vi "Array of params to string.vi"(11 "Array":string[](array[string])) -> (3 "String":string)   [LabVIEW 2019, in "STAV lib.lvlib"]
uses:
  STAV lib.lvlib
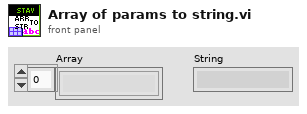
[diagram p1: front panel]
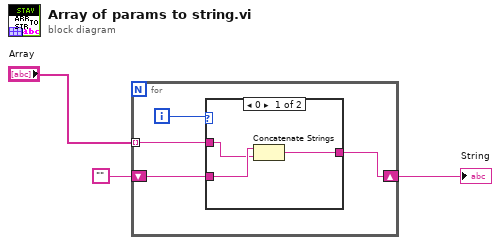
[diagram p0: block diagram]
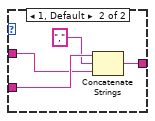
[diagram p2: hidden frame]
diagram:
  n1 = for {
    tunnel: "Array" -> [w6] mode=indexing
    shift-right: [w5] -> w3
    shift-left: "" -> [w7]
    i -> [w4]
    n2 = case shown="0" w4 {
      tunnel: w7 -> [w10 w14]
      tunnel: w6 -> [w9 w13]
      tunnel: [w8 w11] -> w5
      frame 0 {
        n3 = Concatenate Strings(w10, w9) -> (w8:string)
      }
      frame 1, Default {
        n4 = Concatenate Strings(w14, "," ("string"), w13) -> (w11:string)
      }
    }
  }
  "String" <- w3
